vi "调整窗口.vi"(8 "error in (no error)":errorcluster caption="错误输入（无错误）", 10 "前面板范围":T1 caption="窗口范围", 11 "程序响应 输入":refnum<class "程序响应.lvclass">) -> (0 "error out":errorcluster caption="错误输出", 3 "程序响应 输出":refnum<class "程序响应.lvclass">)   [LabVIEW 2018, in "程序响应.lvlib" / "程序响应.lvclass"]
uses:
  <vilib>/Utility/miscctls.llb/LVRectTypeDef.ctl
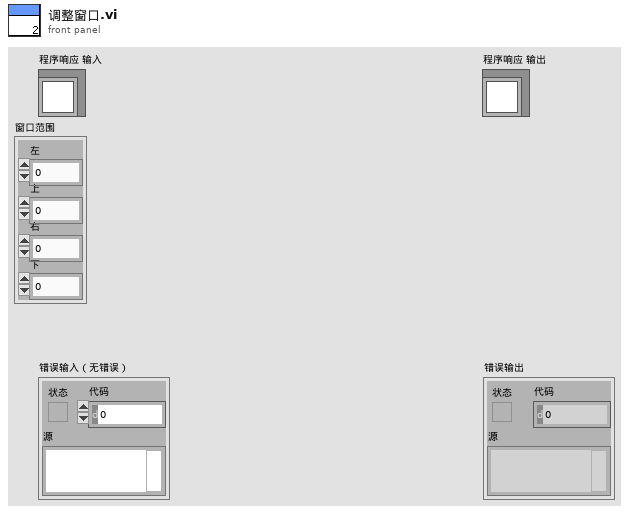
[diagram p1: front panel]
types:
  T1 = typedef "LVRectTypeDef.ctl" = cluster{"Left":i16, "Top":i16, "Right":i16, "Bottom":i16}
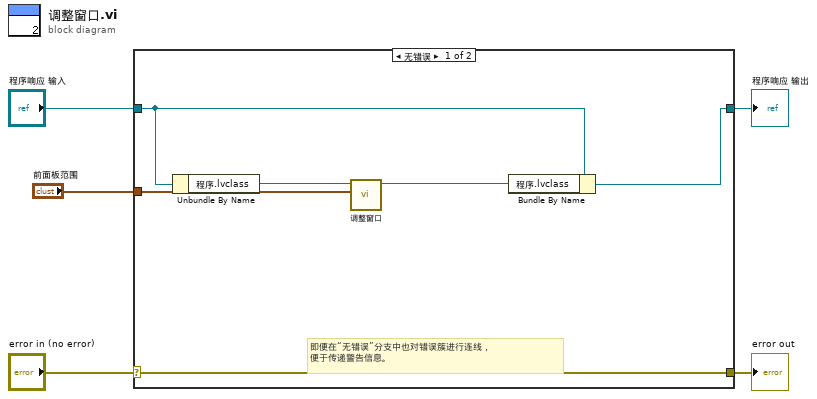
[diagram p0: block diagram]
diagram:
  n1 = case shown="无错误" "error in (no error)" {
    selector: "error in (no error)" -> [w11 w13]
    tunnel: [w11 w13] -> w4
    tunnel: [w6 w12] -> w2
    tunnel: "程序响应 输入" -> [w8 w12]
    tunnel: "前面板范围" -> [w10 _]
    frame No Error {
      # "即便在“无错误”分支中也对错误簇进行连线，\n便于传递警告信息。"
      n2 = Unbundle By Name(w8) -> ("程序.lvclass"=w9:refnum<class "程序.lvclass">)
      n3 = call-dynamic "调整窗口.vi"("前面板范围"=w10, "程序 输入"=w9) -> ("程序 输出"=w7:refnum<class "程序.lvclass">)  [unwired: 8 in, 1 out]
      n4 = Bundle By Name(cluster=w8, "程序.lvclass"=w7) -> (w6:refnum<class "程序响应.lvclass">)
    }
    frame Error {
    }
  }
  "error out" <- w4
  "程序响应 输出" <- w2
